vi "2algarismos.vi"(1 "entrada":string) -> (0 "saida":string)   [LabVIEW 2012]
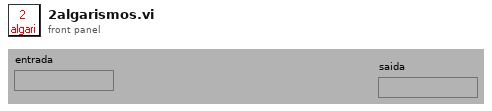
[diagram p1: front panel]
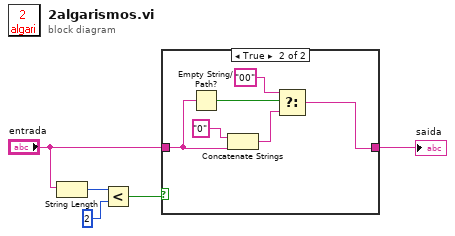
[diagram p0: block diagram]
diagram:
  n1 = String Length(string="entrada") -> (length=w5:i32)
  n2 = Less?(x=w5, y=2) -> (x < y?=w3:bool)
  n3 = case shown="True" w3 {
    tunnel: "entrada" -> [w6 w11]
    tunnel: [w6 w8] -> w1
    frame False {
    }
    frame True {
      n4 = Empty String/Path?(string/path=w11) -> (empty?=w10:bool)
      n5 = Concatenate Strings("0", w11) -> (w9:string)
      n6 = Select(t="00", s=w10, f=w9) -> (s? t:f=w8:string)
    }
  }
  "saida" <- w1
